vi "Example - Multiple On-Off.vi"() -> ()   [LabVIEW 2017]
uses:
  cDAQ/Digital Output/DO_class/DO.lvclass
panel:
  in  "DO On-Off":bool
  out "DO Channel Status":bool[](array[boolean])
  in  "DO Status To Set":bool[](array[boolean])
  in  "DO Channel Number (Zero Based)":i32[](array[numeric])
  in  "Quit Program":bool
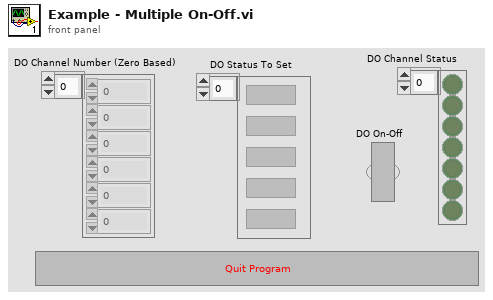
[diagram p1: front panel]
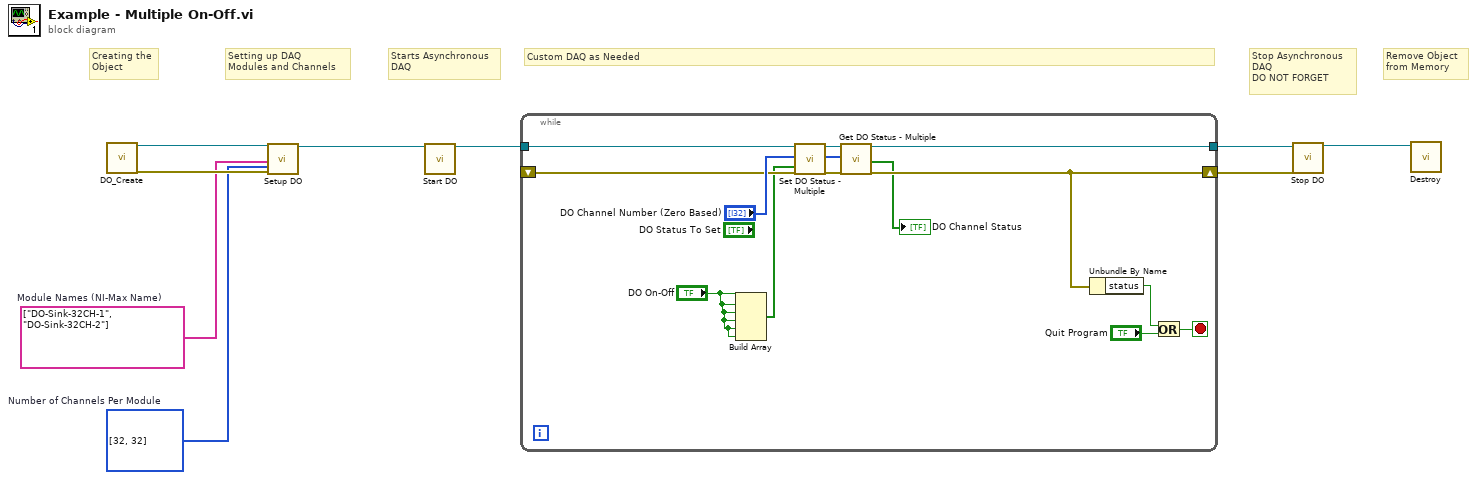
[diagram p0: block diagram]
diagram:
  w6 = u32[] [32, 32]  # Number of Channels Per Module
  w7 = string[] ["DO-Sink-32CH-1", "DO-Sink-32CH-2"]  # Module Names (NI-Max Name)
  # "Custom DAQ as Needed"
  # "Remove Object\nfrom Memory"
  # "Stop Asynchronous\nDAQ\nDO NOT FORGET"
  # "Creating the\nObject"
  # "Setting up DAQ\nModules and Channels"
  # "Starts Asynchronous\nDAQ"
  n1 = call "DO_Create.vi"() -> ("reference out"=w9:refnum<class "DO.lvclass">, "error out"=w8:errorcluster)  [unwired: 18 in]
  n2 = call "Setup DO.vi"("reference in"=w9, "Module Names (NI-MAX Alias)"=w7, "Number of Channels Per Module"=w6, "error in (no error)"=w8) -> ("reference out"=w5:refnum<class "DO.lvclass">)  [unwired: 14 in, 1 out]
  n3 = call-dynamic "Start DO.vi"("reference in"=w5) -> ("reference out"=w2:refnum<class "DO.lvclass">)  [unwired: 17 in, 1 out]
  n4 = while {
    tunnel: w2 -> [w23]
    tunnel: [w21] -> w3
    shift-right: [w17] -> w1
    shift-left: _ -> [w19]
    stop <- w14 stop-if-true
    n5 = Build Array("DO On-Off", "DO On-Off", "DO On-Off", "DO On-Off", "DO On-Off", "DO On-Off") -> (w11:bool[])
    n6 = call-dynamic "Set DO Status - Multiple.vi"("reference in"=w23, "DO Channel Number (Zero Based)"="DO Channel Number (Zero Based)", "DO Status To Set"=w11, "error in (no error)"=w19) -> ("reference out"=w22:refnum<class "DO.lvclass">, "DO Channel Number (Zero Based) OUT"=w13:i32[], "error out"=w18:errorcluster)  [unwired: 13 in]
    n7 = call-dynamic "Get DO Status - Multiple.vi"("reference in"=w22, "DO Channel Numbers (Zero Based)"=w13, "error in (no error)"=w18) -> ("reference out"=w21:refnum<class "DO.lvclass">, "DO Channel Status"=→"DO Channel Status":bool[], "error out"=w17:errorcluster)  [unwired: 14 in]
    n8 = Unbundle By Name(w17) -> ("status"=w16:bool)
    n9 = Or(x=w16, y="Quit Program") -> (x .or. y?=w14:bool)
  }
  n10 = call-dynamic "Stop DO.vi"("reference in"=w3, "error in (no error)"=w1) -> ("reference out"=w4:refnum<class "DO.lvclass">)  [unwired: 16 in, 1 out]
  n11 = call-dynamic "Destroy.vi"("reference in"=w4) -> ()  [unwired: 17 in, 2 out]
